vi "SafeParse_Double.vi"() -> ()   [LabVIEW 2019]
panel:
  in  "Parameter Num":i32
  in  "Parameter Array":string[](array[string])
  in  "vmin":dbl=-1.0
  in  "vmax":dbl=1.0
  out "Value":dbl
  out "Parsing Error":errorcluster
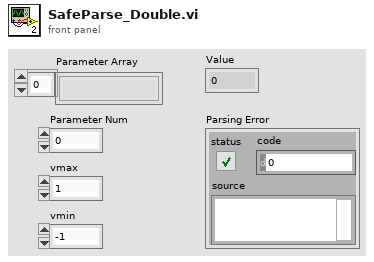
[diagram p1: front panel]
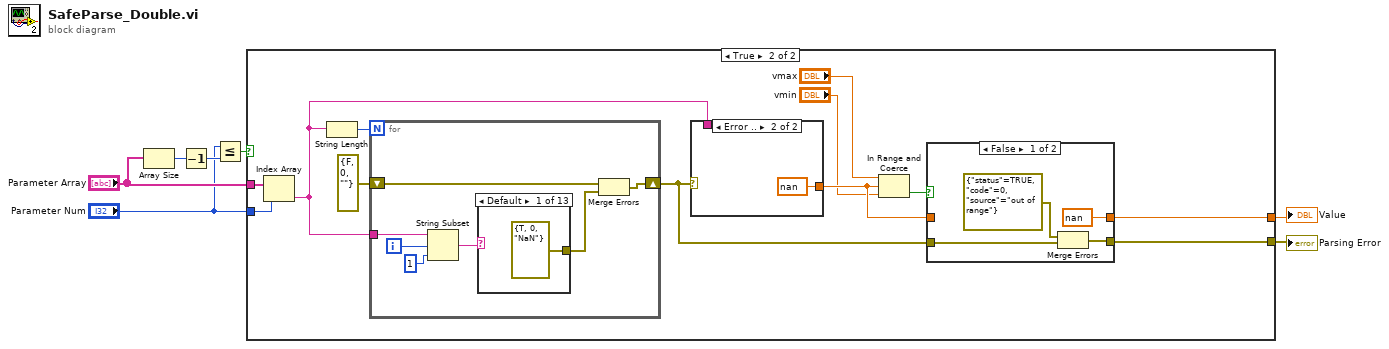
[diagram p0: block diagram]
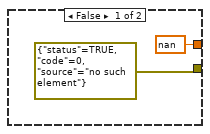
[diagram p2: hidden frame]
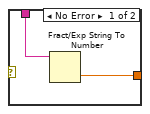
[diagram p4: hidden frame]
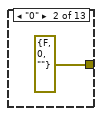
[diagram p5: hidden frame]
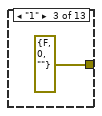
[diagram p6: hidden frame]
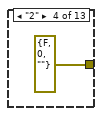
[diagram p7: hidden frame]
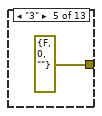
[diagram p8: hidden frame]
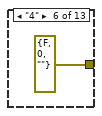
[diagram p9: hidden frame]
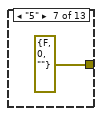
[diagram p10: hidden frame]
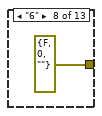
[diagram p11: hidden frame]
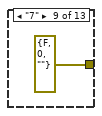
[diagram p12: hidden frame]
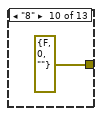
[diagram p13: hidden frame]
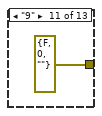
[diagram p14: hidden frame]
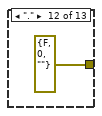
[diagram p15: hidden frame]
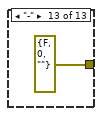
[diagram p16: hidden frame]
diagram:
  n1 = Array Size(array="Parameter Array") -> (size(s)=w6:i32)
  n2 = Decrement(x=w6) -> (x-1=w5:i32)
  n3 = Less Or Equal?(x="Parameter Num", y=w5) -> (x <= y?=w1:bool)
  n4 = case shown="True" w1 {
    tunnel: "Parameter Array" -> [_ w13]
    tunnel: "Parameter Num" -> [_ w12]
    tunnel: [nan w11] -> w3
    tunnel: [errorcluster {"status"=TRUE, "code"=0, "source"="no such element"} ("error constant") w10] -> w2
    frame False {
    }
    frame True {
      n5 = Index Array(array=w13, index=w12) -> (element=w14:string)
      n6 = String Length(string=w14) -> (length=w20:i32)
      n7 = for {
        N: w20 -> [_]
        shift-right: [w36] -> w17
        shift-left: errorcluster {"status"=FALSE, "code"=0, "source"=""} ("error constant") -> [w37]
        tunnel: w14 -> [w35]
        i -> [w33]
        n8 = String Subset(string=w35, offset (0)=w33, length (rest)=1 ("length (rest)")) -> (substring=w32:string)
        n9 = case shown="Default" w32 {
          tunnel: [errorcluster {"status"=TRUE, "code"=0, "source"="NaN"} ("error constant") errorcluster {"status"=FALSE, "code"=0, "source"=""} ("error constant") errorcluster {"status"=FALSE, "code"=0, "source"=""} ("error constant") errorcluster {"status"=FALSE, "code"=0, "source"=""} ("error constant") errorcluster {"status"=FALSE, "code"=0, "source"=""} ("error constant") errorcluster {"status"=FALSE, "code"=0, "source"=""} ("error constant") errorcluster {"status"=FALSE, "code"=0, "source"=""} ("error constant") errorcluster {"status"=FALSE, "code"=0, "source"=""} ("error constant") errorcluster {"status"=FALSE, "code"=0, "source"=""} ("error constant") errorcluster {"status"=FALSE, "code"=0, "source"=""} ("error constant") errorcluster {"status"=FALSE, "code"=0, "source"=""} ("error constant") errorcluster {"status"=FALSE, "code"=0, "source"=""} ("error constant") errorcluster {"status"=FALSE, "code"=0, "source"=""} ("error constant")] -> w31
          frame Default {
          }
          frame "0" {
          }
          frame "1" {
          }
          frame "2" {
          }
          frame "3" {
          }
          frame "4" {
          }
          frame "5" {
          }
          frame "6" {
          }
          frame "7" {
          }
          frame "8" {
          }
          frame "9" {
          }
          frame "." {
          }
          frame "-" {
          }
        }
        n10 = Merge Errors(w37, w31) -> (w36:errorcluster)
      }
      n11 = case shown="Error .." w17 {
        tunnel: w14 -> [w29 _]
        tunnel: [w28 nan] -> w18
        frame No Error {
          n12 = Fract/Exp String To Number(string=w29) -> (number=w28:dbl)  [unwired: 3 in, 1 out]
        }
        frame Error {
        }
      }
      n13 = In Range and Coerce(upper limit="vmax", x=w18, lower limit="vmin") -> (In Range?=w19:bool)  [unwired: 1 out]
      n14 = case shown="False" w19 {
        tunnel: w18 -> [_ w27]
        tunnel: [nan w27] -> w11
        tunnel: w17 -> [w24 w26]
        tunnel: [w23 w26] -> w10
        frame False {
          n15 = Merge Errors(errorcluster {"status"=TRUE, "code"=0, "source"="out of range"} ("error constant"), w24) -> (w23:errorcluster)
        }
        frame True {
        }
      }
    }
  }
  "Value" <- w3
  "Parsing Error" <- w2
